vi "HFRR ADV v020 new software.vi"() -> ()   [LabVIEW 2025] (continued)
            n1439 = formula code="// --- INTERNAL VARIABLE DECLARATIONS ---\nint i = 0;\nint k = 0;\nint start_idx = -1;\nint end_idx = -1;\nint phase = 0;\nint sign0 = 1;\nint sign1 = 1;\nint ch0_val = 0;   \nint ch1_val = 0;   \nfloat ch0_raw = 0.0;\nfloat ch1_raw = 0.0;\nfloat temp0 = 0.0;\nfloat temp1 = 0.0;\nfloat ch0_clean = 0.0;\nfloat ch1_clean = 0.0;\n\n// Initialize output variables to current shift register states right away\nout_LVDT_Min_V = in_LVDT_Min_V;\nout_LVDT_Max_V = in_LVDT_Max_V;\nout_LVDT_P2P_V = in_LVDT_P2P_V;\nout_Piezo_P2P = in_Piezo_P2P;\nout_Friction_N = in_Friction_N;\nout_COF = in_COF;\nwindow_ready = 0;\n\n// --- STEP 1: PARSE EVERY STRING IN THE BYTE ARRAY ---\nif (array_size > 2) {\n    for (i = 0; i < array_size - 1; i++) {\n        if (raw_bytes[i] == 42) { // '*' character detected\n            start_idx = i;\n        }\n        \n        // Match standard delimiter sequence \";&\" or end window character\n        if (raw_bytes[i] == 59 && raw_bytes[i+1] == 38 && start_idx != -1) { \n            end_idx = i;\n            ch0_val = 0;\n            ch1_val = 0;\n            sign0 = 1;\n            sign1 = 1;\n            phase = 0; \n\n            for (k = start_idx + 1; k < end_idx; k++) {\n                if (raw_bytes[k] == 45) { // '-' sign\n                    if (phase == 0) sign0 = -1;\n                    else sign1 = -1;\n                }\n                else if (raw_bytes[k] == 43) { // '+' sign\n                    if (phase == 0) sign0 = 1;\n                    else sign1 = 1;\n                }\n                else if (raw_bytes[k] == 59) { // ';' delimiter\n                    phase = 1; \n                }\n                else if (raw_bytes[k] >= 48 && raw_bytes[k] <= 57) { // Numeric ASCII digits\n                    if (phase == 0) {\n                        ch0_val = (ch0_val * 10) + (raw_bytes[k] - 48);\n                    } else {\n                        ch1_val = (ch1_val * 10) + (raw_bytes[k] - 48);\n                    }\n                }\n            }\n\n            // FIXED: Implicit type conversion by multiplying with a float literal\n            ch0_raw = ch0_val * sign0 * 1.0;\n            ch1_raw = ch1_val * sign1 * 1.0;\n\n            // --- STEP 2: 3-SAMPLE MEDIAN FILTER ---\n            m0_2 = m0_1; m0_1 = m0_0; m0_0 = ch0_raw;\n            float s0_0 = m0_0; float s0_1 = m0_1; float s0_2 = m0_2;\n            if (s0_0 > s0_1) { temp0 = s0_0; s0_0 = s0_1; s0_1 = temp0; }\n            if (s0_1 > s0_2) { temp0 = s0_1; s0_1 = s0_2; s0_2 = temp0; }\n            if (s0_0 > s0_1) { temp0 = s0_0; s0_0 = s0_1; s0_1 = temp0; }\n            ch0_clean = s0_1;\n\n            m1_2 = m1_1; m1_1 = m1_0; m1_0 = ch1_raw;\n            float s1_0 = m1_0; float s1_1 = m1_1; float s1_2 = m1_2;\n            if (s1_0 > s1_1) { temp1 = s1_0; s1_0 = s1_1; s1_1 = temp1; }\n            if (s1_1 > s1_2) { temp1 = s1_1; s1_1 = s1_2; s1_2 = temp1; }\n            if (s1_0 > s1_1) { temp1 = s1_0; s1_0 = s1_1; s1_1 = temp1; }\n            ch1_clean = s1_1;\n\n            // --- STEP 3: EXPONENTIAL FILTER ---\n            if (ch0_filt == 0.0) ch0_filt = ch0_clean;\n            if (ch1_filt == 0.0) ch1_filt = ch1_clean;\n\n            ch0_filt = ch0_filt + (ch0_clean - ch0_filt) * 0.125;\n            ch1_filt = ch1_filt + (ch1_clean - ch1_filt) * 0.125;\n\n            // --- STEP 4: MIN/MAX WINDOW CONTINUOUS ACCUMULATION ---\n            if (ch0_filt > max_ch0) max_ch0 = ch0_filt;\n            if (ch0_filt < min_ch0) min_ch0 = ch0_filt;\n            if (ch1_filt > max_ch1) max_ch1 = ch1_filt;\n            if (ch1_filt < min_ch1) min_ch1 = ch1_filt;\n\n            start_idx = -1; \n        }\n    }\n}\n\n// --- STEP 5: WINDOW EVALUATION ENGINE ---\nif (((current_time_ms - start_time_ms) >= 50) && (min_ch0 < 9000000.0) && (max_ch0 > -9000000.0)) {\n    window_ready = 1;\n\n    // Linear Bit-to-Voltage Transformations\n    out_LVDT_Min_V = (min_ch0 * VREF) / 8388607.0;\n    out_LVDT_Max_V = (max_ch0 * VREF) / 8388607.0;\n    out_LVDT_P2P_V = out_LVDT_Max_V - out_LVDT_Min_V;\n\n    // Piezo scaling calculations\n    out_Piezo_P2P = max_ch1 - min_ch1;\n    out_Friction_N = out_Piezo_P2P * PIEZO_CAL_FACTOR;\n    out_COF = out_Friction_N / NORMAL_FORCE;\n\n    // Reset tracking targets to extreme boundaries safely\n    min_ch0 = 9999999.0;\n    max_ch0 = -9999999.0;\n    min_ch1 = 9999999.0;\n    max_ch1 = -9999999.0;\n\n    start_time_ms = current_time_ms;\n}"("raw_bytes"=w1738, "array_size"=w1737, "VREF"="VREF", "PIEZO_CAL_FACTOR"="PIEZO_CAL_FACTOR", "NORMAL_FORCE"="NORMAL_FORCE", "min_ch0"=w1733, "max_ch0"=w1732, "min_ch1"=w1731, "max_ch1"=w1730, "current_time_ms"=w1725, "start_time_ms"=w1724, "ch0_filt"=w1722, "ch1_filt"=w1721, "m0_0"=w1718, "m0_1"=w1717, "m0_2"=w1716, "m1_0"=w1715, "m1_1"=w1714, "m1_2"=w1713, "in_LVDT_Min_V"=w1706, "in_LVDT_Max_V"=w1699, "in_LVDT_P2P_V"=w1698, "in_Piezo_P2P"=w1697, "in_Friction_N"=w1696, "in_COF"=w1695) -> ("window_ready"=→"Valid_data":dbl, "out_LVDT_Min_V"=w1705:dbl, "out_LVDT_Max_V"=w1704:dbl, "out_LVDT_P2P_V"=w1703:dbl, "out_Piezo_P2P"=w1702:dbl, "out_Friction_N"=w1701:dbl, "out_COF"=w1700:dbl, "min_ch0"=w1729:dbl, "max_ch0"=w1728:dbl, "min_ch1"=w1727:dbl, "max_ch1"=w1726:dbl, "start_time_ms"=w1723:u32, "ch0_filt"=w1720:dbl, "ch1_filt"=w1719:dbl, "m0_0"=w1712:dbl, "m0_1"=w1711:dbl, "m0_2"=w1710:dbl, "m1_0"=w1709:dbl, "m1_1"=w1708:dbl, "m1_2"=w1707:dbl)
            "LVDT MIN" <- w1705
            "LVDT MAX" <- w1704
            "LVDT Peak" <- w1703
            "pizo raw" <- w1702
            "Friction" <- w1701
            "cof" <- w1700
          }
        }
      }
      frame Error {
      }
    }
    n1440 = Wait (ms)(milliseconds to wait=u32 1) -> ()  [unwired: 1 out]
    n1441 = local read "Quit"() -> (w1634:bool)
  }
  n1442 = disable-structure shown="Disabled" {
    disable-tunnel: errorcluster {"status"=TRUE, "code"=0, "source"="Init"} ("error IO") -> [w1761 _]
    disable-tunnel: [w1759 _] -> w48
    frame Disabled {
      n1443 = while {
        shift-right: [w1777] -> w1763
        shift-left: _ -> [w1768]
        shift-right: [w1776] -> w1762
        shift-left: w1761 -> [w1770]
        tunnel: [w1765] -> w1759
        tunnel: [w1775] -> _
        i -> [w1775]
        stop <- w1765 stop-if-true
        n1444 = local read "Port 1a"() -> (w1771:bool)
        n1445 = local read "Port 3"() -> (w1772:bool)
        n1446 = local read "Com Port 1"() -> (w1769:refnum<visa-resource-name>)
        n1447 = Or(x=w1772, y=w1771) -> (x .or. y?=w1774:bool)
        n1448 = Unbundle(w1770) -> ("status"=→"Port 3":bool)  [unwired: 2 out]
        n1449 = Not Equal?(x=w1769, y=w1768) -> (x != y?=w1766:bool)
        n1450 = case shown="True" w1774 {
          frame False {
            w1780 = TRUE ("Visible")
            n1451 = property on="Port 1a" class="Bool (strict)"("Visible"=w1780) -> ()  [unwired: 2 in, 2 out]
            n1452 = property on="Port 3" class="Bool (strict)"("Visible"=w1780) -> ()  [unwired: 2 in, 2 out]
          }
          frame True {
            w1781 = TRUE ("Visible")
            n1453 = property on="Port 1a" class="Bool (strict)"("Visible"=w1781) -> ()  [unwired: 2 in, 2 out]
            n1454 = property on="Port 3" class="Bool (strict)"("Visible"=w1781) -> ()  [unwired: 2 in, 2 out]
          }
        }
        n1455 = Wait (ms)(milliseconds to wait=u32 40) -> ()  [unwired: 1 out]
        n1456 = case shown="True" w1766 {
          tunnel: [w1778 errorcluster {"status"=TRUE, "code"=0, "source"="Init"} ("error out")] -> w1767
          tunnel: w1770 -> [w1778 _]
          frame False {
          }
          frame True {
          }
        }
        "error out 11" <- w1767
        n1457 = case shown="No Error" w1767 {
          selector: w1767 -> [w1788 w1806]
          tunnel: [w1791 w1810] -> w1777
          tunnel: [w1790 w1804] -> w1776
          tunnel: w1768 -> [w1789 w1808]
          frame No Error {
            n1458 = property class="Instr"(reference=w1789, error in=w1788) -> (reference out=w1786:refnum<visa-resource-name>, error out=w1787:errorcluster, "Serial Settings:Number of Bytes at Serial Port"=w1783:u32)
            n1459 = Greater?(x=w1783, y=u32 5) -> (0:w1782:bool)
            n1460 = Not(x=w1782) -> (.not. x?=→"Port 1a":bool)
            n1461 = while {
              tunnel: [w1799] -> w1790
              tunnel: [w1798] -> w1791
              tunnel: w1787 -> [w1797]
              tunnel: w1786 -> [w1796]
              stop <- TRUE stop-if-true
              n1462 = property class="Instr" props=["Serial Settings:Number of Bytes at Serial Port"](reference=w1796, error in=w1797) -> (reference out=w1801:refnum<visa-resource-name>, error out=w1800:errorcluster)  [unwired: 1 out]
              n1463 = VISA Read(VISA resource name=w1801, byte count=u32 50, error in (no error)=w1800) -> (VISA resource name out=w1798:refnum<visa-resource-name>, read buffer=→"UNI READ":string, error out=w1799:errorcluster)  [unwired: 1 out]
              n1464 = Wait (ms)(milliseconds to wait=u32 5) -> ()  [unwired: 1 out]
            }
          }
          frame Error {
            w1816 = u16 0 items=["None", "XON/XOFF", "RTS/CTS", "XON/XOFF & RTS/CTS", "DTR/DSR", "XON/XOFF & DTR/DSR"] ("flow control (0:none)  2")
            w1814 = u16 10 items=["1.0"=10, "1.5"=15, "2.0"=20] ("stop bits 2")
            w1812 = u16 0 items=["None", "Odd", "Even", "Mark", "Space"] ("parity 2")
            w1813 = u32 10000  # timeout (10sec)
            n1465 = VISA Close(VISA resource name=w1808, error in (no error)=w1806) -> (error out=w1809:errorcluster)
            n1466 = local write "Port 1a"(FALSE ("Port 1a")) -> ()
            n1467 = local read "Com Port 1"() -> (w1803:refnum<visa-resource-name>)
            n1468 = call <vilib>:"Clear Errors.vi"("error in (no error)"=w1809) -> ("error out"=w1807:errorcluster)  [unwired: 5 in, 1 out]
            n1469 = call-poly "VISA Configure Serial Port"("VISA resource name"=w1803, "timeout (10sec)"=w1813, "baud rate (9600)"=u32 250000 ("baud rate  2"), "data bits (8)"=u16 8 ("data bits  2"), "parity (0:none)"=w1812, "error in (no error)"=w1807, "stop bits (10: 1 bit)"=w1814, "flow control (0:none)"=w1816) -> ("VISA resource name out"=w1817:refnum<visa-resource-name>, "error out"=w1818:errorcluster)  [unwired: 6 in]
            n1470 = flat-sequence {
              tunnel: w1817 -> [w1820]
              tunnel: w1818 -> [w1819]
              tunnel: [w1820] -> w1810
              tunnel: [w1819] -> w1804
              frame #0 {
                n1471 = Wait (ms)(milliseconds to wait=u32 50) -> ()  [unwired: 1 out]
              }
            }
            "Residual Uno" <- ""
            "Port 1 Error" <- w1804
          }
        }
        n1472 = local read "Quit"() -> (w1765:bool)
        "Error Uno" <- w1770
      }
      n1473 = VISA Close(VISA resource name=w1763, error in (no error)=w1762) -> (error out=w1760:errorcluster)
      n1474 = call <vilib>:"Clear Errors.vi"("error in (no error)"=w1760) -> ()  [unwired: 5 in, 2 out]
    }
    frame Enabled {
    }
  }
  n1475 = while {
    stop <- w1831 stop-if-true
    # "V0OLTAGE TO STROKE (peice vise calibration)"
    n1476 = local read "LVDT MIN"() -> (w1822:dbl)
    n1477 = Wait (ms)(milliseconds to wait=u32 10) -> ()  [unwired: 1 out]
    n1478 = local read "LVDT Peak"() -> (w1823:dbl)
    n1479 = formula code="// Dynamic Parameterized Linear Interpolation Node\n// Inputs: vpp_val, voltages (Array), distances (Array)\n// Outputs: stroke\n\nint i = 0;\nint segments = 11; // 12 points make 11 interpolation segments\n\n// 1. Lower Boundary Clamp\nif (vpp_val <= voltages[0]) {\n    stroke = distances[0];\n}\n// 2. Upper Boundary Clamp\nelse if (vpp_val >= voltages[segments]) {\n    stroke = distances[segments];\n}\n// 3. Dynamic Segment Search Loop\nelse {\n    stroke = distances[0]; // Fallback baseline\n    for (i = 0; i < segments; i++) {\n        if (vpp_val >= voltages[i] && vpp_val <= voltages[i+1]) {\n            // Standard linear interpolation formula using array lookups\n            stroke = distances[i] + (vpp_val - voltages[i]) * (distances[i+1] - distances[i]) / (voltages[i+1] - voltages[i]);\n            break; // Segment found, safely exit the loop\n        }\n    }\n}"("vpp_val"=w1823, "voltages"="calibration values", "distances"="STROKE") -> ("stroke"=→"LVDT STROKE":dbl)
    n1480 = local read "Calibration Tare Value"() -> (w1827:dbl)
    n1481 = local read "Calibration Tare"() -> (w1825:bool)
    n1482 = Subtract(x=w1822, y=w1827) -> (x-y=→"LVDT STROKE  Calibration":dbl)
    n1483 = case shown="True" w1825 {
      selector: w1825 -> [_ w1833]
      tunnel: w1822 -> [_ w1834]
      frame False {
      }
      frame True {
        n1484 = Not(x=w1833) -> (.not. x?=w1832:bool)
        n1485 = local write "Calibration Tare"(w1832) -> ()
        "Calibration Tare Value" <- w1834
      }
    }
    n1486 = local read "Quit"() -> (w1831:bool)
  }
  n1487 = while {
    stop <- w1854 stop-if-true
    n1488 = call <vilib>:"High Resolution Polling Wait.vi"("seconds to wait"=0.02) -> ()  [unwired: 10 in, 1 out]
    n1489 = local read "Due read"() -> (w1852:string)
    n1490 = Spreadsheet String To Array(delimiter (Tab)=";", format string="", spreadsheet string=w1852, array type (2D Dbl)=string[] []) -> (array=w1849:string[])
    n1491 = Fract/Exp String To Number(string=w1849) -> (number=w1848:dbl[])  [unwired: 3 in, 1 out]
    n1492 = Index Array(array=w1848) -> (element #1=→"Sample Temperature":dbl, element #2=→"Target Sample Temperature":dbl, element #3=→"Current Duty Cycle":dbl, element #4=→"Ambient Temperature":dbl, element #5=→"Dac Status":dbl, element #6=→"Vpp":dbl, element #7=→"Active Error Code":dbl, element #8=→"Kp":dbl, element #9=→"Ki":dbl, element #10=→"Kd":dbl, element #11=→"SampleRaw":dbl, element #12=→"AmbRaw":dbl)  [unwired: 12 in]
    n1493 = local read "Quit"() -> (w1854:bool)
  }
  n1494 = while {
    shift-right: [w1868] -> w43
    shift-left: _ -> [w1859]
    shift-right: [w1867] -> w42
    shift-left: errorcluster {"status"=FALSE, "code"=0, "source"="Init"} ("error out") -> [w1861]
    tunnel: [w1856] -> w47
    tunnel: [w1866] -> _
    i -> [w1866]
    stop <- w1856 stop-if-true
    n1495 = local read "Com Port 2"() -> (w1860:refnum<visa-resource-name>)
    n1496 = local read "Port 2a"() -> (w1862:bool)
    n1497 = Unbundle(w1861) -> ("status"=→"Port 4":bool)  [unwired: 2 out]
    n1498 = call <vilib>:"High Resolution Polling Wait.vi"("seconds to wait"=0.02) -> ()  [unwired: 10 in, 1 out]
    n1499 = local read "Port 4"() -> (w1863:bool)
    n1500 = Not Equal?(x=w1860, y=w1859) -> (x != y?=w1858:bool)
    n1501 = Or(x=w1863, y=w1862) -> (x .or. y?=w1865:bool)
    n1502 = case shown="False" w1865 {
      frame False {
        w1871 = TRUE ("Visible")
        n1503 = property on="Port 2a" class="Bool (strict)"("Visible"=w1871) -> ()  [unwired: 2 in, 2 out]
        n1504 = property on="Port 4" class="Bool (strict)"("Visible"=w1871) -> ()  [unwired: 2 in, 2 out]
      }
      frame True {
        w1872 = TRUE ("Visible")
        n1505 = property on="Port 2a" class="Bool (strict)"("Visible"=w1872) -> ()  [unwired: 2 in, 2 out]
        n1506 = property on="Port 4" class="Bool (strict)"("Visible"=w1872) -> ()  [unwired: 2 in, 2 out]
      }
    }
    n1507 = case shown="True" w1858 {
      tunnel: [w1869 errorcluster {"status"=TRUE, "code"=0, "source"="Init"} ("error out")] -> w1857
      tunnel: w1861 -> [w1869 _]
      frame False {
      }
      frame True {
      }
    }
    n1508 = case shown="No Error" w1857 {
      selector: w1857 -> [w1885 w1916]
      tunnel: [w1878 w1921] -> w1868
      tunnel: [w1886 w1914] -> w1867
      tunnel: w1859 -> [w1887 w1919]
      frame No Error {
        n1509 = property class="Instr" props=["Serial Settings:Number of Bytes at Serial Port"](reference=w1887, error in=w1885) -> (reference out=w1879:refnum<visa-resource-name>, error out=w1884:errorcluster)  [unwired: 1 out]
        n1510 = while {
          tunnel: [w1895] -> w1880
          tunnel: [w1894] -> w1881
          tunnel: w1884 -> [w1893]
          tunnel: w1879 -> [w1892]
          tunnel: [w1891] -> _
          i -> [w1891]
          stop <- TRUE stop-if-true
          n1511 = property class="Instr" props=["Serial Settings:Number of Bytes at Serial Port"](reference=w1892, error in=w1893) -> (reference out=w1897:refnum<visa-resource-name>, error out=w1896:errorcluster)  [unwired: 1 out]
          n1512 = VISA Read(VISA resource name=w1897, byte count=u32 1000, error in (no error)=w1896) -> (VISA resource name out=w1894:refnum<visa-resource-name>, read buffer=→"Due read":string, error out=w1895:errorcluster)  [unwired: 1 out]
        }
        n1513 = local read "Command"() -> (w1877:string)
        n1514 = call <vilib>:"Trim Whitespace.vi"("string"=w1877) -> ("trimmed string"=w1876:string)  [unwired: 1 in]
        n1515 = Not Equal?(x=w1876, y="") -> (x != y?=w1882:bool)
        n1516 = VISA Flush I/O Buffer(VISA resource name=w1881) -> (VISA resource name out=w1874:refnum<visa-resource-name>, error out=→"error out 10":errorcluster)  [unwired: 2 in]
        n1517 = case shown="True" w1882 {
          tunnel: w1874 -> [w1899 w1904]
          tunnel: [w1899 w1908] -> w1878
          tunnel: w1880 -> [w1898 w1903]
          tunnel: [w1898 w1906] -> w1886
          tunnel: w1876 -> [_ w1902]
          tunnel: [_ w1905] -> _
          frame False {
            # "DATA  WRITE LOOP"
          }
          frame True {
            n1518 = Concatenate Strings(w1902, "\r\n") -> (w1901:string)
            n1519 = VISA Write(VISA resource name=w1904, write buffer=w1901, error in (no error)=w1903) -> (VISA resource name out=w1908:refnum<visa-resource-name>, return count=w1905:u32, error out=w1907:errorcluster)
            n1520 = flat-sequence {
              tunnel: w1907 -> [w1910]
              tunnel: [w1910] -> w1906
              frame #0 {
                n1521 = local write "Command"("" ("Command")) -> ()
                n1522 = Wait (ms)(milliseconds to wait=u32 5) -> ()  [unwired: 1 out]
              }
            }
          }
        }
        "Port 2a" <- TRUE ("Port 2a")
      }
      frame Error {
        w1927 = u16 0 items=["None", "XON/XOFF", "RTS/CTS", "XON/XOFF & RTS/CTS", "DTR/DSR", "XON/XOFF & DTR/DSR"] ("flow control (0:none)  2")
        w1925 = u16 10 items=["1.0"=10, "1.5"=15, "2.0"=20] ("stop bits 2")
        w1923 = u16 0 items=["None", "Odd", "Even", "Mark", "Space"] ("parity 2")
        w1924 = u32 10000  # timeout (10sec)
        n1523 = VISA Clear(VISA resource name=w1919, error in (no error)=w1916) -> (VISA resource name out=w1918:refnum<visa-resource-name>, error out=w1917:errorcluster)
        n1524 = VISA Close(VISA resource name=w1918, error in (no error)=w1917) -> (error out=w1920:errorcluster)
        n1525 = call <vilib>:"Clear Errors.vi"("error in (no error)"=w1920) -> ()  [unwired: 5 in, 2 out]
        n1526 = local write "Port 2a"(FALSE ("Port 2a")) -> ()
        n1527 = local read "Com Port 2"() -> (w1913:refnum<visa-resource-name>)
        "visa due" <- w1913
        n1528 = call-poly "VISA Configure Serial Port"("VISA resource name"=w1913, "timeout (10sec)"=w1924, "baud rate (9600)"=u32 250000 ("baud rate  2"), "data bits (8)"=u16 8 ("data bits  2"), "parity (0:none)"=w1923, "stop bits (10: 1 bit)"=w1925, "flow control (0:none)"=w1927) -> ("VISA resource name out"=w1928:refnum<visa-resource-name>, "error out"=w1929:errorcluster)  [unwired: 7 in]
        n1529 = flat-sequence {
          tunnel: w1928 -> [w1931]
          tunnel: w1929 -> [w1930]
          tunnel: [w1931] -> w1921
          tunnel: [w1930] -> w1914
          frame #0 {
            n1530 = Wait (ms)(milliseconds to wait=u32 50) -> ()  [unwired: 1 out]
          }
        }
        "Residual Due" <- ""
        "Port 2 Error" <- w1914
      }
    }
    n1531 = local read "Quit"() -> (w1856:bool)
    "Error Due" <- w1861
  }
  n1532 = local write "FRICVALZ"(0.0 ("FRICVALZ")) -> ()
  n1533 = property on="RUN" class="Bool (strict)"("Visible"=TRUE) -> ()  [unwired: 2 in, 2 out]
  n1534 = while {
    tunnel: [w1948] -> _
    tunnel: [w1933] -> w57
    i -> [w1948]
    stop <- w1933 stop-if-true
    n1535 = local read "conststatus"() -> (w1937:dbl)
    n1536 = local read "Main Tab"() -> (w1935:T2)
    n1537 = local read "EDIT"() -> (w1954:bool)
    n1538 = local read "Rate"() -> (w1953:dbl)
    n1539 = case shown="True" w1954 {
      tunnel: [FALSE TRUE] -> w1940
      frame False {
      }
      frame True {
      }
    }
    n1540 = property on="Time slide" class="Slide (strict)"("Scale.Range:Maximum"=2500.0) -> ()  [unwired: 2 in, 2 out]
    n1541 = Equal?(x=w1935, y=T27."About" ("Main Tab")) -> (x = y?=w1946:bool)
    n1542 = Equal?(x=w1937, y=0.0) -> (x = y?=w1938:bool)
    n1543 = Divide(x=1.0, y=w1953) -> (x/y=w1949:dbl)
    "Time 2" <- w1949
    n1544 = case shown="True" w1938 {
      frame False {
      }
      frame True {
        # "C:\\WinDucom\\calibrate WO 2391.dcf"
        n1545 = local write "Lan flag"(22) -> ()
        n1546 = local write "conststatus"(10.0 ("rpm value : 2")) -> ()
        n1547 = String To Path(string="C:\\LAB-IQ\\calibrate WO 2465.dcf") -> (path=w1960:path)
        n1548 = Open/Create/Replace File "Open File"(file path (use dialog)=w1960) -> (refnum out=w1958:refnum<file>)  [unwired: 5 in, 2 out]
        n1549 = for {
          N: 23 -> [_]
          tunnel: w1958 -> [w1969]
          i -> [w1963]
          (unwired) TRUE ("line mode (F)")
          n1550 = Read from Text File "Read File"(file (use dialog)=w1969) -> (text=w1968:string)  [unwired: 3 in, 3 out]
          n1551 = Match Pattern(string=w1968, regular expression="]") -> (after substring=w1966:string)  [unwired: 1 in, 3 out]
          n1552 = String Subset(string=w1968, offset (0)=5, length (rest)=10 ("length (rest)")) -> (substring=w1961:string)
          n1553 = Fract/Exp String To Number(string=w1961) -> (number=w1962:dbl)  [unwired: 3 in, 1 out]
          n1554 = Match Pattern(string=w1966, regular expression="-") -> (before substring=w1964:string)  [unwired: 1 in, 3 out]
          n1555 = case shown="4" w1963 {
            tunnel: w1962 -> [w1972 w1973 w1974 w1975 _ _ _ w1980 w1981 _ w1982 w1983 w1984 w1985 w1986 w1987 _ w1988 w1989 _ _ _ _ _]
            tunnel: w1964 -> [_ _ _ _ w1976 w1977 w1978 _ _ _ _ _ _ _ _ _ _ _ _ w1990 w1991 w1992 w1993 _]
            frame 0 {
              n1556 = local write "FRIC. FORCE :"(w1972) -> ()
            }
            frame 1 {
              n1557 = local write "TEMPERATURE :"(w1973) -> ()
            }
            frame 2 {
              n1558 = local write "HUMIDITY:"(w1974) -> ()
            }
            frame 3 {
              n1559 = local write "AIR TEMPERATURE :"(w1975) -> ()
            }
            frame 4 {
              n1560 = local write "Com Port 1"(w1976) -> ()
            }
            frame 5 {
              n1561 = local write "Com Port 2"(w1977) -> ()
              n1562 = local write "visa due"(w1977) -> ()
            }
            frame 6 {
              n1563 = String To Path(string=w1978) -> (path=w1979:path)
              n1564 = local write "File Path"(w1979) -> ()
              "String" <- w1978
            }
            frame 7 {
              n1565 = local write "DISPLACEMENT :"(w1980) -> ()
            }
            frame 8 {
              n1566 = local write "STROKE GAIN :"(w1981) -> ()
            }
            frame 9 {
            }
            frame 10 {
              n1567 = local write "Language Selection"(w1982) -> ()
            }
            frame 11 {
              n1568 = local write "CH-POWER +"(w1983) -> ()
            }
            frame 12 {
              n1569 = local write "CH-POWER -"(w1984) -> ()
            }
            frame 13 {
              n1570 = local write "CH-HEATER"(w1985) -> ()
            }
            frame 14 {
              n1571 = local write "CH-HUMIDITY WET"(w1986) -> ()
            }
            frame 15 {
              n1572 = local write "CH-HUMIDITY DRY"(w1987) -> ()
            }
            frame 16 {
            }
            frame 17 {
              n1573 = local write "AIR TEMP INTERCEPT:"(w1988) -> ()
            }
            frame 18 {
              n1574 = local write "TEMP INTERCEPT:"(w1989) -> ()
            }
            frame 21 {
              n1575 = local write "S.NO"(w1990) -> ()
            }
            frame 22 {
              n1576 = local write "Com Port 3"(w1991) -> ()
            }
            frame 20 {
              n1577 = local write "Camera Port :"(w1992) -> ()
            }
            frame 19 {
              n1578 = local write "C3 :"(w1993) -> ()
            }
            frame 23, Default {
            }
          }
        }
      }
    }
    n1579 = Select(t=u32 2500 ("milliseconds to wait"), s=w1946, f=u32 500 ("milliseconds to wait")) -> (s? t:f=w1944:u32)
    n1580 = Multiply(x=w1949, y=w1944) -> (x*y=w1951:dbl)
    n1581 = property on="Time slide" class="Slide (strict)"("Visible"=w1940) -> ()  [unwired: 2 in, 2 out]
    n1582 = call "Elapsed Time2"("Time Target (s)"=w1951, "Auto Reset"=TRUE) -> ("Time has Elapsed"=w1941:bool)  [unwired: 10 in, 7 out]
    n1583 = case shown="True" w1941 {
      frame False {
      }
      frame True {
        n1584 = stacked-sequence {
          frame #0 {
            # "DATA PROCESSING"
            # "115 mV/N"
            n1585 = local read "Sample Temperature"() -> (w1996:dbl)
            n1586 = local read "RH Numeric:"() -> (w2003:dbl)
            n1587 = local read "HUMIDITY:"() -> (w2004:dbl)
            n1588 = local read "FRICVALZ"() -> (w2015:dbl)
            n1589 = local read "Friction"() -> (w1999:dbl)
            n1590 = Multiply(x=w2003, y=w2004) -> (x*y=→"Humidity ( %RH )" →"Hum" →"Hum 2":dbl)
            n1591 = call <vilib>:"Mean PtByPt.vi"("x"=w1996, "sample length"=100) -> ("mean"=w1995:dbl)  [unwired: 2 in, 1 out]
            "TEMP 2" <- w1995
            "TEMP 3" <- w1995
            n1592 = Subtract(x=w1999, y=w2015) -> (x-y=w2010:dbl)
            "FF 2" <- w2010
            "FF 4" <- w2010
            n1593 = local read "Ambient Temperature"() -> (→"AIR TEMP":dbl)
            n1594 = local read "TEMP"() -> (w2014:dbl)
            n1595 = local write "FF 3"(w2010) -> ()
            n1596 = Compound Arithmetic op=OR("FRICVALZ 4", "FRICVALZ 3", "FRICVALZ 2") -> (w2006:bool)
            n1597 = case shown="True" w2006 {
              tunnel: w1999 -> [_ w2021]
              frame False {
              }
              frame True {
                w2020 = FALSE ("FRICVALZ")
                n1598 = local write "FRICVALZ 3"(w2020) -> ()
                n1599 = local write "FRICVALZ 2"(w2020) -> ()
                n1600 = local write "FRICVALZ 4"(w2020) -> ()
                "FRICVALZ" <- w2021
              }
            }
            n1601 = Not A Number/Path/Refnum?(number/path/refnum=w2014) -> (NaN/Path/Refnum?=w2013:bool)
            n1602 = Not A Number/Path/Refnum?(number/path/refnum=w2010) -> (NaN/Path/Refnum?=w2012:bool)
            n1603 = Divide(x=w2010, y=1.96) -> (x/y=w2007:dbl)
            n1604 = Compound Arithmetic op=OR(w2013, w2012) -> (w2011:bool)
            n1605 = Not A Number/Path/Refnum?(number/path/refnum=w2007) -> (NaN/Path/Refnum?=w2008:bool)
            n1606 = case shown="True" w2011 {
              frame False {
              }
              frame True {
                n1607 = local write "TEMP"(0.0 ("TEMP")) -> ()
                n1608 = local write "FF 2"(0.0 ("FF 2")) -> ()
                n1609 = local write "reinit"(TRUE ("reinit")) -> ()
              }
            }
            n1610 = local write "TEMP"(w1995) -> ()
            n1611 = Select(t=0.0, s=w2008, f=w2007) -> (s? t:f=w1998:dbl)
            "COF 2" <- w1998
            n1612 = local write "COF 3"(w1998) -> ()
          }
        }
      }
    }
    n1613 = Wait (ms)(milliseconds to wait=u32 50) -> ()  [unwired: 1 out]
    n1614 = local read "Quit"() -> (w1933:bool)
    "Rate" <- 2500.0 ("No of Samples")
  }
  n1615 = while {
    tunnel: w60 -> [_]
    tunnel: [w2048] -> _
    tunnel: [w2024] -> w59
    i -> [w2048]
    stop <- w2024 stop-if-true
    # "C:\\LAB-IQ-NXT\\Scar View.exe"
    n1616 = local read "OK Button 16"() -> (w2037:bool)
    n1617 = local read "Main Tab"() -> (w2030:T2)
    n1618 = local read "service 3"() -> (w2031:bool)
    n1619 = local read "OPEN 6"() -> (w2033:bool)
    n1620 = local read "EDIT 2"() -> (w2035:bool)
    n1621 = flat-sequence {
      frame #0 {
        n1622 = local read "SAVE 2"() -> (w2650:bool)
        n1623 = stacked-sequence {
          frame #0 {
            n1624 = local read "EDIT"() -> (w2704:bool)
            n1625 = case shown="True" w2704 {
              tunnel: [u8 2 ("Disabled") u8 0 ("Disabled")] -> _
              frame False {
                w2706 = FALSE
                n1626 = local write "Password"("") -> ()
                n1627 = property on="SrvM CP" class="Bool (strict)"("Visible"=w2706) -> ()  [unwired: 2 in, 2 out]
                n1628 = property on="message" class="Str"("Visible"=w2706) -> ()  [unwired: 2 in, 2 out]
                n1629 = local write "x = y?"(w2706) -> ()
                n1630 = property on="Password" class="Str"("Visible"=w2706) -> ()  [unwired: 2 in, 2 out]
                n1631 = property on="ENTER THE NEW PASSWORD" class="Str"("Visible"=w2706) -> ()  [unwired: 2 in, 2 out]
                n1632 = property on="ENTER CURRENT PASSWORD" class="Str"("Visible"=w2706) -> ()  [unwired: 2 in, 2 out]
                n1633 = local write "SrvM CP"(w2706) -> ()
              }
              frame True {
                w2709 = TRUE
                n1634 = property on="SrvM CP" class="Bool (strict)"("Visible"=w2709) -> ()  [unwired: 2 in, 2 out]
                n1635 = property on="Password" class="Str"("Visible"=w2709) -> ()  [unwired: 2 in, 2 out]
              }
            }
            "dipl pwd" <- "@143$\n" ("dipl pwd")
          }
          frame #1 {
            # "Gain password"
            n1636 = String To Byte Array(string="ENTER CURRENT PASSWORD") -> (unsigned byte array=w2714:u8[])
            n1637 = Search 1D Array(1D array=w2714, element=u8 10) -> (index of element=w2717:i32)  [unwired: 1 in]
            n1638 = Index Array(array=w2714, index=w2717) -> (element=w2713:u8)
            n1639 = Equal?(x=w2713, y=10) -> (x = y?=w2711:bool)
            n1640 = case shown="True" w2711 {
              frame False {
                n1641 = property on="ENTER THE NEW PASSWORD" class="Str"("Visible"=FALSE) -> ()  [unwired: 2 in, 2 out]
              }
              frame True {
                # "password"
                # "change password logic"
                n1642 = local read "ENTER CURRENT PASSWORD"() -> (w2730:string)
                n1643 = local read "dipl pwd"() -> (w2724:string)
                n1644 = String To Byte Array(string=w2730) -> (unsigned byte array=w2732:u8[])
                n1645 = String To Byte Array(string=w2724) -> (unsigned byte array=w2725:u8[])
                n1646 = Array Size(array=w2732) -> (size(s)=w2729:i32)
                n1647 = Array Size(array=w2725) -> (size(s)=w2727:i32)
                n1648 = for {
                  N: w2729 -> [_]
                  tunnel: w2732 -> [w2756]
                  tunnel: [w2754] -> w2733 mode=indexing
                  tunnel: w2729 -> [w2748]
                  i -> [w2749]
                  n1649 = Decrement(x=w2748) -> (x-1=w2746:i32)
                  n1650 = Equal?(x=w2749, y=w2746) -> (x = y?=w2747:bool)
                  n1651 = Index Array(array=w2756, index=w2749) -> (element=w2750:u8)
                  n1652 = Number To Decimal String(number=w2750) -> (decimal integer string=w2755:string)  [unwired: 1 in]
                  n1653 = Select(t="", s=w2747, f="\r") -> (s? t:f=w2752:string)
                  n1654 = Concatenate Strings(w2755, w2752) -> (w2754:string)
                }
                n1655 = for {
                  N: w2727 -> [_]
                  tunnel: w2725 -> [w2744]
                  tunnel: [w2742] -> w2726 mode=indexing
                  tunnel: w2727 -> [w2739]
                  i -> [w2740]
                  n1656 = Decrement(x=w2739) -> (x-1=w2738:i32)
                  n1657 = Equal?(x=w2740, y=w2738) -> (x = y?=w2737:bool)
                  n1658 = Index Array(array=w2744, index=w2740) -> (element=w2743:u8)
                  n1659 = Number To Decimal String(number=w2743) -> (decimal integer string=w2741:string)  [unwired: 1 in]
                  n1660 = Select(t="", s=w2737, f="\r") -> (s? t:f=w2734:string)
                  n1661 = Concatenate Strings(w2741, w2734) -> (w2742:string)
                }
                n1662 = local read "string"() -> (w2731:string)
                n1663 = Concatenate Strings(w2726) -> (w2720:string)
                n1664 = Concatenate Strings(w2731) -> (w2728:string)
                n1665 = Concatenate Strings(w2733) -> (w2721:string)
                n1666 = Equal?(x=w2721, y=w2728) -> (x = y?=w2723:bool)
                n1667 = Equal?(x=w2721, y=w2720) -> (x = y?=w2719:bool)
                n1668 = Or(x=w2723, y=w2719) -> (x .or. y?=w2722:bool)
                n1669 = case shown="True" w2722 {
                  frame False {
                  }
                  frame True {
                    n1670 = property on="ENTER THE NEW PASSWORD" class="Str"("Visible"=TRUE) -> ()  [unwired: 2 in, 2 out]
                  }
                }
              }
            }
          }
          frame #2 {
            n1671 = String To Byte Array(string="ENTER THE NEW PASSWORD") -> (unsigned byte array=w2759:u8[])
            n1672 = Search 1D Array(1D array=w2759, element=u8 10) -> (index of element=w2763:i32)  [unwired: 1 in]
            n1673 = Index Array(array=w2759, index=w2763) -> (element=w2761:u8)
            n1674 = Equal?(x=w2761, y=10) -> (x = y?=w2758:bool)
            n1675 = case shown="False" w2758 {
              frame False {
              }
              frame True {
                n1676 = local write "EDIT"(FALSE) -> ()
                n1677 = local write "SrvM CP"(FALSE) -> ()
                n1678 = local read "ENTER THE NEW PASSWORD"() -> (w2766:string)
                n1679 = String To Byte Array(string=w2766) -> (unsigned byte array=w2771:u8[])
                n1680 = Array Size(array=w2771) -> (size(s)=w2768:i32)
                n1681 = for {
                  N: w2768 -> [_]
                  tunnel: w2771 -> [w2784]
                  tunnel: [w2781] -> w2773 mode=indexing
                  tunnel: w2768 -> [w2776]
                  i -> [w2774]
                  n1682 = Decrement(x=w2776) -> (x-1=w2777:i32)
                  n1683 = Equal?(x=w2774, y=w2777) -> (x = y?=w2778:bool)
                  n1684 = Index Array(array=w2784, index=w2774) -> (element=w2783:u8)
                  n1685 = Number To Decimal String(number=w2783) -> (decimal integer string=w2782:string)  [unwired: 1 in]
                  n1686 = Select(t="", s=w2778, f="\r") -> (s? t:f=w2775:string)
                  n1687 = Concatenate Strings(w2782, w2775) -> (w2781:string)
                }
                n1688 = local read "file path"() -> (w2765:path)
                n1689 = Concatenate Strings(w2773) -> (w2767:string)
                n1690 = Delete(path (use dialog)=w2765) -> (deleted path=w2769:path)  [unwired: 4 in, 2 out]
                n1691 = call <vilib>:"Write Characters To File.vi"("append to file? (new file:F)"=FALSE, "character string"=w2767, "file path (dialog if empty)"=w2769) -> ()  [unwired: 2 in, 1 out]
              }
            }
          }
          frame #3 {
            n1692 = case shown="True" "SrvM CP" {
              frame False {
                w2787 = ""
                n1693 = local write "ENTER CURRENT PASSWORD"(w2787) -> ()
                n1694 = local write "ENTER THE NEW PASSWORD"(w2787) -> ()
                n1695 = property on="ENTER CURRENT PASSWORD" class="Str"("Visible"=FALSE) -> ()  [unwired: 2 in, 2 out]
              }
              frame True {
                n1696 = property on="ENTER THE NEW PASSWORD" class="Str"() -> ("Visible"=w2788:bool)  [unwired: 2 in, 2 out]
                n1697 = Not(x=w2788) -> (.not. x?=w2789:bool)
                n1698 = property on="ENTER CURRENT PASSWORD" class="Str"("Visible"=w2789) -> ()  [unwired: 2 in, 2 out]
              }
            }
          }
          frame #4 {
            n1699 = String To Byte Array(string="Password") -> (unsigned byte array=w2796:u8[])
            n1700 = Search 1D Array(1D array=w2796, element=u8 10) -> (index of element=w2794:i32)  [unwired: 1 in]
            n1701 = Index Array(array=w2796, index=w2794) -> (element=w2795:u8)
            n1702 = Equal?(x=w2795, y=10) -> (x = y?=w2791:bool)
            n1703 = case shown="True" w2791 {
              frame False {
              }
              frame True {
                # "password"
                # "password"
                n1704 = local read "Password"() -> (w2809:string)
                n1705 = String To Byte Array(string=w2809) -> (unsigned byte array=w2812:u8[])
                n1706 = String To Byte Array(string="@143$\n") -> (unsigned byte array=w2798:u8[])
                n1707 = Array Size(array=w2812) -> (size(s)=w2807:i32)
                n1708 = Array Size(array=w2798) -> (size(s)=w2803:i32)
                n1709 = for {
                  N: w2807 -> [_]
                  tunnel: w2812 -> [w2846]
                  tunnel: [w2844] -> w2813 mode=indexing
                  tunnel: w2807 -> [w2841]
                  i -> [w2842]
                  n1710 = Decrement(x=w2841) -> (x-1=w2840:i32)
                  n1711 = Index Array(array=w2846, index=w2842) -> (element=w2845:u8)
                  n1712 = Equal?(x=w2842, y=w2840) -> (x = y?=w2839:bool)
                  n1713 = Number To Decimal String(number=w2845) -> (decimal integer string=w2843:string)  [unwired: 1 in]
                  n1714 = Select(t="", s=w2839, f="\r") -> (s? t:f=w2836:string)
                  n1715 = Concatenate Strings(w2843, w2836) -> (w2844:string)
                }
                n1716 = for {
                  N: w2803 -> [_]
                  tunnel: w2798 -> [w2857]
                  tunnel: [w2855] -> w2801 mode=indexing
                  tunnel: w2803 -> [w2852]
                  i -> [w2853]
                  n1717 = Decrement(x=w2852) -> (x-1=w2851:i32)
                  n1718 = Index Array(array=w2857, index=w2853) -> (element=w2856:u8)
                  n1719 = Equal?(x=w2853, y=w2851) -> (x = y?=w2850:bool)
                  n1720 = Number To Decimal String(number=w2856) -> (decimal integer string=w2854:string)  [unwired: 1 in]
                  n1721 = Select(t="", s=w2850, f="\r") -> (s? t:f=w2847:string)
                  n1722 = Concatenate Strings(w2854, w2847) -> (w2855:string)
                }
                n1723 = local read "file path"() -> (w2797:path)
                n1724 = call <vilib>:"Read Characters From File.vi"("file path (dialog if empty)"=w2797) -> ("character string"=w2811:string)  [unwired: 5 in, 3 out]
                "string" <- w2811
                n1725 = flat-sequence {
                  tunnel: [w2814] -> w2808
                  frame #0 {
                    w2814 = ""
                    n1726 = local write "Password"(w2814) -> ()
                  }
                }
                n1727 = Concatenate Strings(w2801) -> (w2802:string)
                n1728 = Concatenate Strings(w2811) -> (w2810:string)
                n1729 = Concatenate Strings(w2813) -> (w2805:string)
                n1730 = Equal?(x=w2805, y=w2810) -> (x = y?=w2800:bool)
                n1731 = Equal?(x=w2805, y=w2802) -> (x = y?=w2806:bool)
                n1732 = Or(x=w2800, y=w2806) -> (x .or. y?=w2799:bool)
                "x = y?" <- w2799
                n1733 = case shown="True" w2799 {
                  selector: w2799 -> [w2816 _]
                  tunnel: w2808 -> [_ _]
                  frame False {
                    n1734 = And(x=w2816, y=TRUE ("Visible")) -> (x .and. y?=w2817:bool)
                    n1735 = property on="message" class="Str"("Visible"=w2817) -> ()  [unwired: 2 in, 2 out]
                  }
                  frame True {
                    n1736 = control-ref of="This VI"() -> (w2828:refnum<vi>)
                    n1737 = property class="VI"(reference=w2828) -> (reference out=w2819:refnum<vi>, error out=w2823:errorcluster, "Panel"=w2827:refnum<vi>)  [unwired: 1 in]
                    n1738 = property on="message" class="Str"("Visible"=FALSE) -> ()  [unwired: 2 in, 2 out]
                    n1739 = property class="Pnl"(reference=w2827, error in=w2823) -> (reference out=w2821:refnum<vi>, error out=w2824:errorcluster, "Panes[]"=w2826:refnum<vi>[])
                    n1740 = for {
                      tunnel: w2826 -> [w2835] mode=indexing
                      tunnel: T21."Always On" ("Horizontal Scrollbar Visibility") -> [w2834]
                      tunnel: w2824 -> [w2831]
                      tunnel: [w2830] -> w2822
                      n1741 = property class="Pane"(reference=w2835, error in=w2831, "HorizScrollbarVisibility"=w2834) -> (reference out=w2832:refnum<vi>, error out=w2833:errorcluster)
                      n1742 = Close Reference(reference=w2832, error in (no error)=w2833) -> (error out=w2830:errorcluster)
                    }
                    n1743 = Close Reference(reference=w2821, error in (no error)=w2822) -> (error out=w2820:errorcluster)
                    n1744 = Close Reference(reference=w2819, error in (no error)=w2820) -> (error out=→"error out 6":errorcluster)
                  }
                }
              }
            }
          }
        }
        n1745 = local read "x = y?"() -> (w2656:bool)
        n1746 = local read "HUMIDITY: 2"() -> (w2658:dbl)
        n1747 = local read "HUMIDITY:"() -> (w2657:dbl)
        n1748 = property on="Port 2 Error" class="Clust (strict)"("Visible"="EDIT") -> ()  [unwired: 2 in, 2 out]
        n1749 = property on="Port 1 Error" class="Clust (strict)"("Visible"="EDIT") -> ()  [unwired: 2 in, 2 out]
        n1750 = case shown="True" "SrvM CP 2" {
          frame False {
          }
          frame True {
            n1751 = local write "SrvM CP 2"(FALSE ("SrvM CP 2")) -> ()
            n1752 = local read "HUMIDITY: 2"() -> (w2697:dbl)
            n1753 = local read "TEMP INTERCEPT: 2"() -> (w2696:dbl)
            n1754 = local read "DISPLACEMENT : 4"() -> (w2700:dbl)
            n1755 = local read "TEMPERATURE : 2"() -> (w2699:dbl)
            n1756 = local read "STROKE GAIN : 2"() -> (w2701:dbl)
            n1757 = local read "FRIC. FORCE : 2"() -> (w2702:dbl)
            n1758 = local read "AIR TEMP INTERCEPT: 2"() -> (w2695:dbl)
            n1759 = local read "AIR TEMPERATURE : 2"() -> (w2698:dbl)
            n1760 = local write "HUMIDITY:"(w2697) -> ()
            n1761 = local write "AIR TEMP INTERCEPT:"(w2696) -> ()
            n1762 = local write "TEMPERATURE :"(w2699) -> ()
            n1763 = local write "FRIC. FORCE :"(w2702) -> ()
            n1764 = local write "STROKE GAIN :"(w2701) -> ()
            n1765 = local write "DISPLACEMENT :"(w2700) -> ()
            n1766 = local write "AIR TEMPERATURE :"(w2698) -> ()
            n1767 = local write "TEMP INTERCEPT:"(w2695) -> ()
          }
        }
        n1768 = Or(x="SAVE", y=w2650) -> (x .or. y?=w2651:bool)
        n1769 = And(x="EDIT", y=w2656) -> (x .and. y?=w2654:bool)
        n1770 = local read "DISPLACEMENT : 4"() -> (w2667:dbl)
        n1771 = local read "TEMPERATURE : 2"() -> (w2665:dbl)
        n1772 = local read "STROKE GAIN : 2"() -> (w2671:dbl)
        n1773 = local read "DISPLACEMENT :"() -> (w2666:dbl)
        n1774 = local read "FRIC. FORCE : 2"() -> (w2674:dbl)
        n1775 = local read "TEMPERATURE :"() -> (w2663:dbl)
        n1776 = local read "STROKE GAIN :"() -> (w2670:dbl)
        n1777 = local read "FRIC. FORCE :"() -> (w2673:dbl)
        n1778 = case shown="True" w2654 {
          tunnel: [u8 2 ("Disabled") u8 0 ("Disabled")] -> w2653
          tunnel: [w3018 TRUE ("Visible")] -> w2652
          frame False {
            w3018 = FALSE ("Visible")
            n1779 = local write "EDIT 2"(w3018) -> ()
          }
          frame True {
          }
        }
        n1780 = case shown="True" w2651 {
          frame False {
          }
          frame True {
            n1781 = stacked-sequence {
              seq-local: [w2866 _ _] -> [_ w3013 _]
              frame #0 {
                (unwired) i16 5 ("precision (6)")
                # "[CH1]    - FF\n[CH2]   - TEMPERATURE\n[CH3]    - Humidity\n[CH4]    - AIR TEMP\n[CH5]\\- Visa Uno\n[CH6] \\- Visa Due\n[CH7]  \\- file path\n[CH8]   - Displacement Gain\n[CHA]   - Stroke Gain\n[CHB]   - Stroke PID Gain\n[CHC]   -Language Selection\n[CHD]   -Power +\n[CHE]   -Power_\n[CHF]   -Heater\n[CHG]   -Humidity Wet\n[CHH]   -Humidity Dry\n[CHI]   -Integral Time"
                n1782 = local read "Language Selection"() -> (w2914:enum16{"English", "Russian"})
                n1783 = local read "CH-HUMIDITY WET"() -> (w2872:u16)
                n1784 = local read "CH-HUMIDITY DRY"() -> (w2869:u16)
                n1785 = local read "STROKE GAIN :"() -> (w2858:dbl)
                n1786 = local read "CH-POWER +"() -> (w2881:u16)
                n1787 = local read "CH-POWER -"() -> (w2878:u16)
                n1788 = local read "CH-HEATER"() -> (w2875:u16)
                n1789 = local read "AIR TEMPERATURE :"() -> (w2861:dbl)
                n1790 = local read "DISPLACEMENT :"() -> (w2859:dbl)
                n1791 = local read "TEMPERATURE :"() -> (w2862:dbl)
                n1792 = local read "FRIC. FORCE :"() -> (w2863:dbl)
                n1793 = local read "HUMIDITY:"() -> (w2860:dbl)
                n1794 = Path To String(path="File Path") -> (string=w2930:string)
                n1795 = Number To Fractional String(number=w2858, width (-)=i16 10 ("precision (6)"), precision (6)=i16 5) -> (F-format string=w2921:string)  [unwired: 1 in]
                n1796 = Number To Fractional String(number=w2914, width (-)=i16 10 ("precision (6)"), precision (6)=i16 5) -> (F-format string=w2910:string)  [unwired: 1 in]
                n1797 = Number To Fractional String(number=w2881, width (-)=i16 10 ("precision (6)"), precision (6)=i16 5) -> (F-format string=w2904:string)  [unwired: 1 in]
                n1798 = Number To Fractional String(number=w2878, width (-)=i16 10 ("precision (6)"), precision (6)=i16 5) -> (F-format string=w2901:string)  [unwired: 1 in]
                n1799 = Number To Fractional String(number=w2875, width (-)=i16 10 ("precision (6)"), precision (6)=i16 5) -> (F-format string=w2896:string)  [unwired: 1 in]
                n1800 = Number To Fractional String(number=w2872, width (-)=i16 10 ("precision (6)"), precision (6)=i16 5) -> (F-format string=w2893:string)  [unwired: 1 in]
                n1801 = Number To Fractional String(number=w2869, width (-)=i16 10 ("precision (6)"), precision (6)=i16 5) -> (F-format string=w2888:string)  [unwired: 1 in]
                n1802 = local read "Com Port 1"() -> (w2865:refnum<visa-resource-name>)
                n1803 = local read "Com Port 2"() -> (w2864:refnum<visa-resource-name>)
                n1804 = Concatenate Strings(w2930, "\\" ("string")) -> (w2929:string)
                n1805 = Number To Fractional String(number=w2863, width (-)=i16 10 ("precision (6)"), precision (6)=i16 5) -> (F-format string=w2962:string)  [unwired: 1 in]
                n1806 = Number To Fractional String(number=w2862, width (-)=i16 10 ("precision (6)"), precision (6)=i16 5) -> (F-format string=w2961:string)  [unwired: 1 in]
                n1807 = Number To Fractional String(number=w2860, width (-)=i16 10 ("precision (6)"), precision (6)=i16 5) -> (F-format string=w2955:string)  [unwired: 1 in]
                n1808 = Number To Fractional String(number=w2861, width (-)=i16 10 ("precision (6)"), precision (6)=i16 5) -> (F-format string=w2949:string)  [unwired: 1 in]
                n1809 = Number To Fractional String(number=w2859, width (-)=i16 10 ("precision (6)"), precision (6)=i16 5) -> (F-format string=w2922:string)  [unwired: 1 in]
                n1810 = Concatenate Strings("[CHA]" ("string"), w2921, "- Stroke Gain" ("string"), "\r") -> (w2915:string)
                n1811 = Concatenate Strings("[CHC]" ("string"), w2910, "-Language Selection" ("string"), "\r") -> (w2907:string)
                n1812 = Concatenate Strings("[CHD]" ("string"), w2904, "-Power +" ("string"), "\r") -> (w2886:string)
                n1813 = Concatenate Strings("[CHG]" ("string"), w2893, "-Humidity Wet" ("string"), "\r") -> (w2883:string)
                n1814 = Concatenate Strings("[CHH]" ("string"), w2888, "-Humidity Dry" ("string"), "\r") -> (w2882:string)
                n1815 = Concatenate Strings("[CH1]" ("string"), w2962, " - FF" ("string"), "\r") -> (w2960:string)
                n1816 = Concatenate Strings("[CH2]" ("string"), w2961, " - TEMPERATURE" ("string"), "\r") -> (w2959:string)
                n1817 = Concatenate Strings("[CH3]" ("string"), w2955, " - Humidity" ("string"), "\r") -> (w2952:string)
                n1818 = Concatenate Strings("[CH4]" ("string"), w2949, " - AIR TEMP" ("string"), "\r") -> (w2945:string)
                n1819 = Concatenate Strings("[CH5]" ("string"), w2865, "- Visa Uno" ("string"), "\r") -> (w2938:string)
                n1820 = Concatenate Strings("[CH6]" ("string"), w2864, "- Visa Due" ("string"), "\r") -> (w2933:string)
                n1821 = Concatenate Strings("[CH7]" ("string"), w2929, "- file path" ("string"), "\r") -> (w2932:string)
                n1822 = Concatenate Strings("[CH8]" ("string"), w2922, "- Displacement Gain" ("string"), "\r") -> (w2925:string)
                n1823 = Concatenate Strings("[CHE]" ("string"), w2901, "-Power_" ("string"), "\r") -> (w2885:string)
                n1824 = Concatenate Strings("[CHF]" ("string"), w2896, "-Heater" ("string"), "\r") -> (w2884:string)
                n1825 = Concatenate Strings(w2960, w2959, w2952, w2945, w2938, w2933, w2932, w2925, w2915, w2907, w2886, w2885, w2884, w2883, w2882) -> (w2866:string)
                "gain" <- w2866
              }
              frame #1 {
                n1826 = local read "Camera Port :"() -> (w2974:string)
                n1827 = local read "C3 :"() -> (w2982:refnum<visa-resource-name>)
                n1828 = local read "TEMP INTERCEPT:"() -> (w2983:dbl)
                n1829 = local read "AIR TEMP INTERCEPT:"() -> (w2984:dbl)
                n1830 = local read "Com Port 3"() -> (w2985:refnum<visa-resource-name>)
                n1831 = Concatenate Strings("[CH8]" ("string"), w2974, "- Visa Camera" ("string"), "\r") -> (w2973:string)
                n1832 = Concatenate Strings("[CH7]" ("string"), w2982, "- Visa Humidity" ("string"), "\r") -> (w2978:string)
                n1833 = Number To Fractional String(number=w2983, width (-)=i16 10 ("precision (6)"), precision (6)=i16 5) -> (F-format string=w3001:string)  [unwired: 1 in]
                n1834 = Concatenate Strings("[CHL]" ("string"), w2985, "- Visa humid" ("string"), "\r") -> (w2988:string)
                n1835 = Number To Fractional String(number=w2984, width (-)=i16 10 ("precision (6)"), precision (6)=i16 5) -> (F-format string=w3008:string)  [unwired: 1 in]
                n1836 = Concatenate Strings("[CHK]" ("string"), w3001, "-TEMP INTERCEPT" ("string"), "\r") -> (w2997:string)
                n1837 = Concatenate Strings("[SNO]" ("string"), "S.NO", "-" ("string"), "\r") -> (w2993:string)
                n1838 = Concatenate Strings("[CHJ]" ("string"), w3008, "-AIR TEMP INTERCEPT" ("string"), "\r") -> (w2998:string)
                n1839 = String To Path(string="C:\\LAB-IQ\\calibrate WO 2465.dcf") -> (path=w2986:path)
                n1840 = Concatenate Strings(w3013, w2998, w2997, w2993, w2988, w2978, w2973) -> (w3012:string)
                n1841 = call <vilib>:"Write Characters To File.vi"("append to file? (new file:F)"=FALSE, "character string"=w3012, "file path (dialog if empty)"=w2986) -> ()  [unwired: 2 in, 1 out]
              }
              frame #2 {
                n1842 = local write "Lan flag"(0.0 ("Lan flag")) -> ()
                n1843 = local write "conststatus"(0.0 ("rpm value : 2")) -> ()
                n1844 = local write "SAVE"(FALSE ("OK Button 14")) -> ()
                n1845 = local write "SAVE 2"(FALSE ("SAVE 2")) -> ()
              }
            }
          }
        }
        n1846 = Subtract(x=w2658, y=w2657) -> (x-y=w2659:dbl)
        n1847 = local read "AIR TEMPERATURE : 2"() -> (w2662:dbl)
        n1848 = local read "AIR TEMPERATURE :"() -> (w2661:dbl)
        n1849 = Divide(x=w2659, y=w2657) -> (x/y=w2681:dbl)
        n1850 = Subtract(x=w2674, y=w2673) -> (x-y=w2672:dbl)
        n1851 = Subtract(x=w2665, y=w2663) -> (x-y=w2664:dbl)
        n1852 = Subtract(x=w2671, y=w2670) -> (x-y=w2669:dbl)
        n1853 = Subtract(x=w2667, y=w2666) -> (x-y=w2668:dbl)
        n1854 = Subtract(x=w2662, y=w2661) -> (x-y=w2660:dbl)
        n1855 = Divide(x=w2672, y=w2673) -> (x/y=w2692:dbl)
        n1856 = Divide(x=w2664, y=w2663) -> (x/y=w2685:dbl)
        n1857 = Divide(x=w2669, y=w2670) -> (x/y=w2689:dbl)
        n1858 = Divide(x=w2668, y=w2666) -> (x/y=w2688:dbl)
        n1859 = Multiply(x=w2681, y=100.0) -> (x*y=→"HUMIDITY  Calibration Error":dbl)
        n1860 = Divide(x=w2660, y=w2661) -> (x/y=w2684:dbl)
        n1861 = Multiply(x=w2692, y=100.0) -> (x*y=→"FRIC. FORCE Calibration Error":dbl)
        n1862 = Multiply(x=w2685, y=100.0) -> (x*y=→"TEMPERATURE  Calibration Error":dbl)
        n1863 = Multiply(x=w2689, y=100.0) -> (x*y=→"STROKE Calibration Error":dbl)
        n1864 = Multiply(x=w2688, y=100.0) -> (x*y=→"DISPLACEMENT  Calibration Error":dbl)
        n1865 = property on="EDIT 2" class="Bool (strict)"("Visible"=w2652) -> ()  [unwired: 2 in, 2 out]
        n1866 = property on="SAVE" class="Bool (strict)"("Visible"=w2652) -> ()  [unwired: 2 in, 2 out]
        n1867 = property on="SrvM CP" class="Bool (strict)"("Disabled"=w2653) -> ()  [unwired: 2 in, 2 out]
        n1868 = property on="visa due" class="CmbBox"("Disabled"=w2653) -> ()  [unwired: 2 in, 2 out]
        n1869 = property on="File Path" class="Path"("Disabled"=w2653) -> ()  [unwired: 2 in, 2 out]
        n1870 = Multiply(x=w2684, y=100.0) -> (x*y=→"AIR TEMPERATURE  Calibration Error":dbl)
        n1871 = property on="Language Selection" class="Enum (strict)"("Visible"=w2652) -> ()  [unwired: 2 in, 2 out]
        n1872 = property on="Tab Control 7" class="TabCtl (strict)"("Disabled"=w2653) -> ()  [unwired: 2 in, 2 out]
        n1873 = property on="AIR TEMP INTERCEPT:" class="DigNum (strict)"("Disabled"=w2653) -> ()  [unwired: 2 in, 2 out]
        n1874 = property on="CH-POWER -" class="DigNum (strict)"("Disabled"=w2653) -> ()  [unwired: 2 in, 2 out]
        n1875 = property on="CH-POWER +" class="DigNum (strict)"("Disabled"=w2653) -> ()  [unwired: 2 in, 2 out]
        n1876 = property on="AIR TEMPERATURE :" class="DigNum (strict)"("Disabled"=w2653) -> ()  [unwired: 2 in, 2 out]
        n1877 = property on="STROKE GAIN :" class="DigNum (strict)"("Disabled"=w2653) -> ()  [unwired: 2 in, 2 out]
        n1878 = property on="SPEED OUT:" class="DigNum (strict)"("Disabled"=w2653) -> ()  [unwired: 2 in, 2 out]
        n1879 = property on="CH-HUMIDITY DRY" class="DigNum (strict)"("Disabled"=w2653) -> ()  [unwired: 2 in, 2 out]
        n1880 = property on="HUMIDITY:" class="DigNum (strict)"("Disabled"=w2653) -> ()  [unwired: 2 in, 2 out]
        n1881 = property on="CH-HUMIDITY WET" class="DigNum (strict)"("Disabled"=w2653) -> ()  [unwired: 2 in, 2 out]
        n1882 = property on="TEMPERATURE :" class="DigNum (strict)"("Disabled"=w2653) -> ()  [unwired: 2 in, 2 out]
        n1883 = property on="DISPLACEMENT :" class="DigNum (strict)"("Disabled"=w2653) -> ()  [unwired: 2 in, 2 out]
        n1884 = property on="CH-HEATER" class="DigNum (strict)"("Disabled"=w2653) -> ()  [unwired: 2 in, 2 out]
        n1885 = property on="TEMP INTERCEPT:" class="DigNum (strict)"("Disabled"=w2653) -> ()  [unwired: 2 in, 2 out]
        n1886 = property on="FRIC. FORCE :" class="DigNum (strict)"("Disabled"=w2653) -> ()  [unwired: 2 in, 2 out]
      }
    }
    n1887 = local read "RUN"() -> (w2047:bool)
    n1888 = local read "RUN"() -> (w2045:bool)
    n1889 = disable-structure shown="Disabled" {
      disable-tunnel: [w2062 _] -> w2028
      disable-tunnel: [w2061 _] -> w2026
      frame Disabled {
        n1890 = local read "Temperature before test"() -> (w2055:dbl)
        n1891 = local read "Temperature after test"() -> (w2068:dbl)
        n1892 = case shown="True" "Save Results" {
          frame False {
          }
          frame True {
            w2084 = "\r"
            n1893 = local write "Save Results"(FALSE ("OK Button 5")) -> ()
            n1894 = local read "Temperature before test"() -> (w2122:dbl)
            n1895 = local read "Temperature after test"() -> (w2124:dbl)
            n1896 = local read "Humidity before test"() -> (w2121:dbl)
            n1897 = local read "Humidity after test"() -> (w2123:dbl)
            n1898 = local read "WS1.4"() -> (w2128:dbl)
            n1899 = local read "AVP"() -> (w2126:dbl)
            n1900 = Number To Fractional String(number=w2128, width (-)=i16 6, precision (6)=i16 1) -> (F-format string=w2088:string)  [unwired: 1 in]
            n1901 = local read "MWSD"() -> (w2125:dbl)
            n1902 = local read "String"() -> (w2117:string)
            n1903 = local read "FILE"() -> (w2120:string)
            n1904 = local read "HCF"() -> (w2127:dbl)
            n1905 = Number To Fractional String(number=w2121, width (-)=i16 6, precision (6)=i16 1) -> (F-format string=w2113:string)  [unwired: 1 in]
            n1906 = Number To Fractional String(number=w2122, width (-)=i16 6, precision (6)=i16 1) -> (F-format string=w2110:string)  [unwired: 1 in]
            n1907 = Number To Fractional String(number=w2123, width (-)=i16 6, precision (6)=i16 1) -> (F-format string=w2106:string)  [unwired: 1 in]
            n1908 = Number To Fractional String(number=w2124, width (-)=i16 6, precision (6)=i16 1) -> (F-format string=w2102:string)  [unwired: 1 in]
            n1909 = Number To Fractional String(number=w2126, width (-)=i16 6, precision (6)=i16 3) -> (F-format string=w2095:string)  [unwired: 1 in]
            n1910 = Concatenate Strings(w2117, w2120) -> (w2139:string)
            n1911 = Number To Fractional String(number=w2125, width (-)=i16 6, precision (6)=i16 1) -> (F-format string=w2099:string)  [unwired: 1 in]
            n1912 = Number To Fractional String(number=w2127, width (-)=i16 6, precision (6)=i16 2) -> (F-format string=w2093:string)  [unwired: 1 in]
            n1913 = Concatenate Strings("(" ("string"), w2088, ")Microns" ("string")) -> (w2087:string)
            n1914 = local read "REMARKS"() -> (w2119:string)
            "REMARKS 2" <- w2119
            n1915 = Concatenate Strings("(" ("string"), w2113, " ) % RH," ("string")) -> (w2114:string)
            n1916 = Concatenate Strings(w2093, ")" ("string")) -> (w2091:string)
            n1917 = Concatenate Strings("(" ("string"), w2110, ")  Deg C ," ("string")) -> (w2109:string)
            n1918 = Concatenate Strings("(" ("string"), w2106, " ) % RH," ("string")) -> (w2105:string)
            n1919 = Concatenate Strings("(" ("string"), w2102, ")  Deg C ," ("string")) -> (w2101:string)
            n1920 = Concatenate Strings("(" ("string"), w2099, ")  Microns," ("string")) -> (w2098:string)
            n1921 = Concatenate Strings("(" ("string"), w2095, ")  kPa," ("string")) -> (w2085:string)
            n1922 = Concatenate Strings(w2139, ".dwm" ("Substring")) -> (w2137:string)
            n1923 = String To Path(string=w2137) -> (path=w2136:path)
            n1924 = Concatenate Strings(w2119, w2084, " Humidity before test= " ("Substring"), w2114, w2084, " Temperature before test = " ("Substring"), w2109, w2084, " Humidity after test= " ("Substring"), w2105, w2084, "Temperature after test = " ("Substring"), w2101, w2084, "MSD = " ("Substring"), w2098, w2084, "  AVP = " ("Substring"), w2085, w2084, "  HCF                     =( " ("Substring"), w2091, w2084, " WS1.4                  = " ("Substring"), w2087, w2084) -> (w2083:string)
            "data" <- w2083
            n1925 = call <vilib>:"Write Characters To File.vi"("append to file? (new file:F)"=FALSE, "character string"=w2083, "file path (dialog if empty)"=w2136) -> ()  [unwired: 2 in, 1 out]
            n1926 = Match Pattern(string=w2083, regular expression="!") -> (after substring=→"export":string)  [unwired: 1 in, 3 out]
          }
        }
        n1927 = Add(x=231.864, y=w2055) -> (x+y=w2052:dbl)
        n1928 = Add(x=231.864, y=w2068) -> (x+y=w2065:dbl)
        n1929 = Divide(x=1705.984, y=w2052) -> (x/y=w2053:dbl)
        n1930 = Divide(x=1705.984, y=w2065) -> (x/y=w2066:dbl)
        n1931 = local read "Humidity before test"() -> (w2057:dbl)
        n1932 = local read "Humidity after test"() -> (w2070:dbl)
        n1933 = Subtract(x=8.017352 ("y"), y=w2053) -> (x-y=w2079:dbl)
        n1934 = Subtract(x=8.017352 ("y"), y=w2066) -> (x-y=w2073:dbl)
        n1935 = expression code="10**y"(w2079) -> (w2059:dbl)
        n1936 = expression code="10**y"(w2073) -> (w2072:dbl)
        n1937 = Multiply(x=w2057, y=w2059) -> (x*y=w2058:dbl)
        n1938 = Multiply(x=w2070, y=w2072) -> (x*y=w2071:dbl)
        n1939 = Divide(x=w2058, y=750.0) -> (x/y=w2074:dbl)
        n1940 = Divide(x=w2071, y=750.0) -> (x/y=w2075:dbl)
        n1941 = Add(x=w2074, y=w2075) -> (x+y=w2076:dbl)
        n1942 = Divide(x=w2076, y=2.0) -> (x/y=w2078:dbl)
        n1943 = local write "AVP"(w2078) -> ()
        n1944 = Subtract(x=1.4, y=w2078) -> (x-y=w2061:dbl)
        n1945 = local read "HCF"() -> (w2062:dbl)
      }
      frame Enabled {
      }
    }
    n1946 = case shown="True" "EDIT 3" {
      frame False {
      }
      frame True {
        n1947 = local write "EDIT 3"(FALSE ("EDIT 3")) -> ()
        n1948 = local write "Main Tab"(T2."About" ("Main Tab")) -> ()
      }
    }
    n1949 = case shown="False" w2047 {
      frame False {
        n1950 = local read "stopT"() -> (w3025:bool)
        n1951 = case shown="True" w3025 {
          frame False {
          }
          frame True {
            n1952 = local write "stopT"(FALSE) -> ()
          }
        }
      }
      frame True {
        "stopT" <- TRUE
      }
    }
